vi "DTMF_RealTimeSignalProcessing_Final_COPY.vi"() -> ()   [LabVIEW 2020]
uses:
  <vilib>/Waveform/WDTOps.llb/WDT Index Channel DBL.vi
  <vilib>/Waveform/WDTOps.llb/WDT Get Waveform Subset DBL.vi
  <vilib>/measure/matone.llb/Extract Single Tone Information 1 Chan.vi
  <vilib>/measure/matone.llb/Extract Multiple Tone Information 1 Chan.vi
  <vilib>/measure/NI_MAPro.lvlib
panel:
  out "FFT spectrum - Complete Signal":cluster{"f0":dbl, "df":dbl, "magnitude":dbl[]}(graph)
  in  "Emergency stop":bool
  out "Time Domain Signal - Complete Signal":dbl(graph)
  in  "Bypasing mode - Loop Timer (ms)":u32(knob)=5 scale=0.0..50.0
  out "Case1 - Time Signal":waveform(dbl)(graph)
  out "Case1 - Spectrum":cluster{"f0":dbl, "df":dbl, "magnitude":dbl[]}(graph)
  out "Lower Frequency":T1(array[cluster]) {"detected phase (deg)" format="%_6g"; "detected amplitude" format="%_6p"; "detected frequency" format="%_6f"}
  out "Case1 Subarray Length":dbl
  out "Case1\nTrigger\nStatus":bool
  out "Higher Frequency":T1(array[cluster]) {"detected phase (deg)" format="%_6g"; "detected amplitude" format="%_6p"; "detected frequency" format="%_6f"}
  out "Case0 Subarray Length":dbl
  out "Case0 Start Index":dbl
  out "Time Domain Signal - Detected Button Presses":dbl(graph)
  in  "Scanning mode - Loop Timer (ms)":u32(knob)=5 scale=0.0..50.0
  out "Total Samples(s)":i32
  out "Case1 Start Index":dbl
  out "Case0 - Time Signal":waveform(dbl)(graph)
  out "Case0 - Spectrum":cluster{"f0":dbl, "df":dbl, "magnitude":dbl[]}(graph)
  out "Case0\nTrigger\nStatus":bool
  out "Iteration#":i32
  out "DTMF Number":string
  in  "Select .wav file":path
  # "This program is for the real time processing of the DTMF signals\nPlease adjust the knobs are increasing the scanning speed"
  # "Case - 0 Scanning mode"
  # "Case - 1 Bypassing mode"
  # "Adjust knobs for scanning speed"
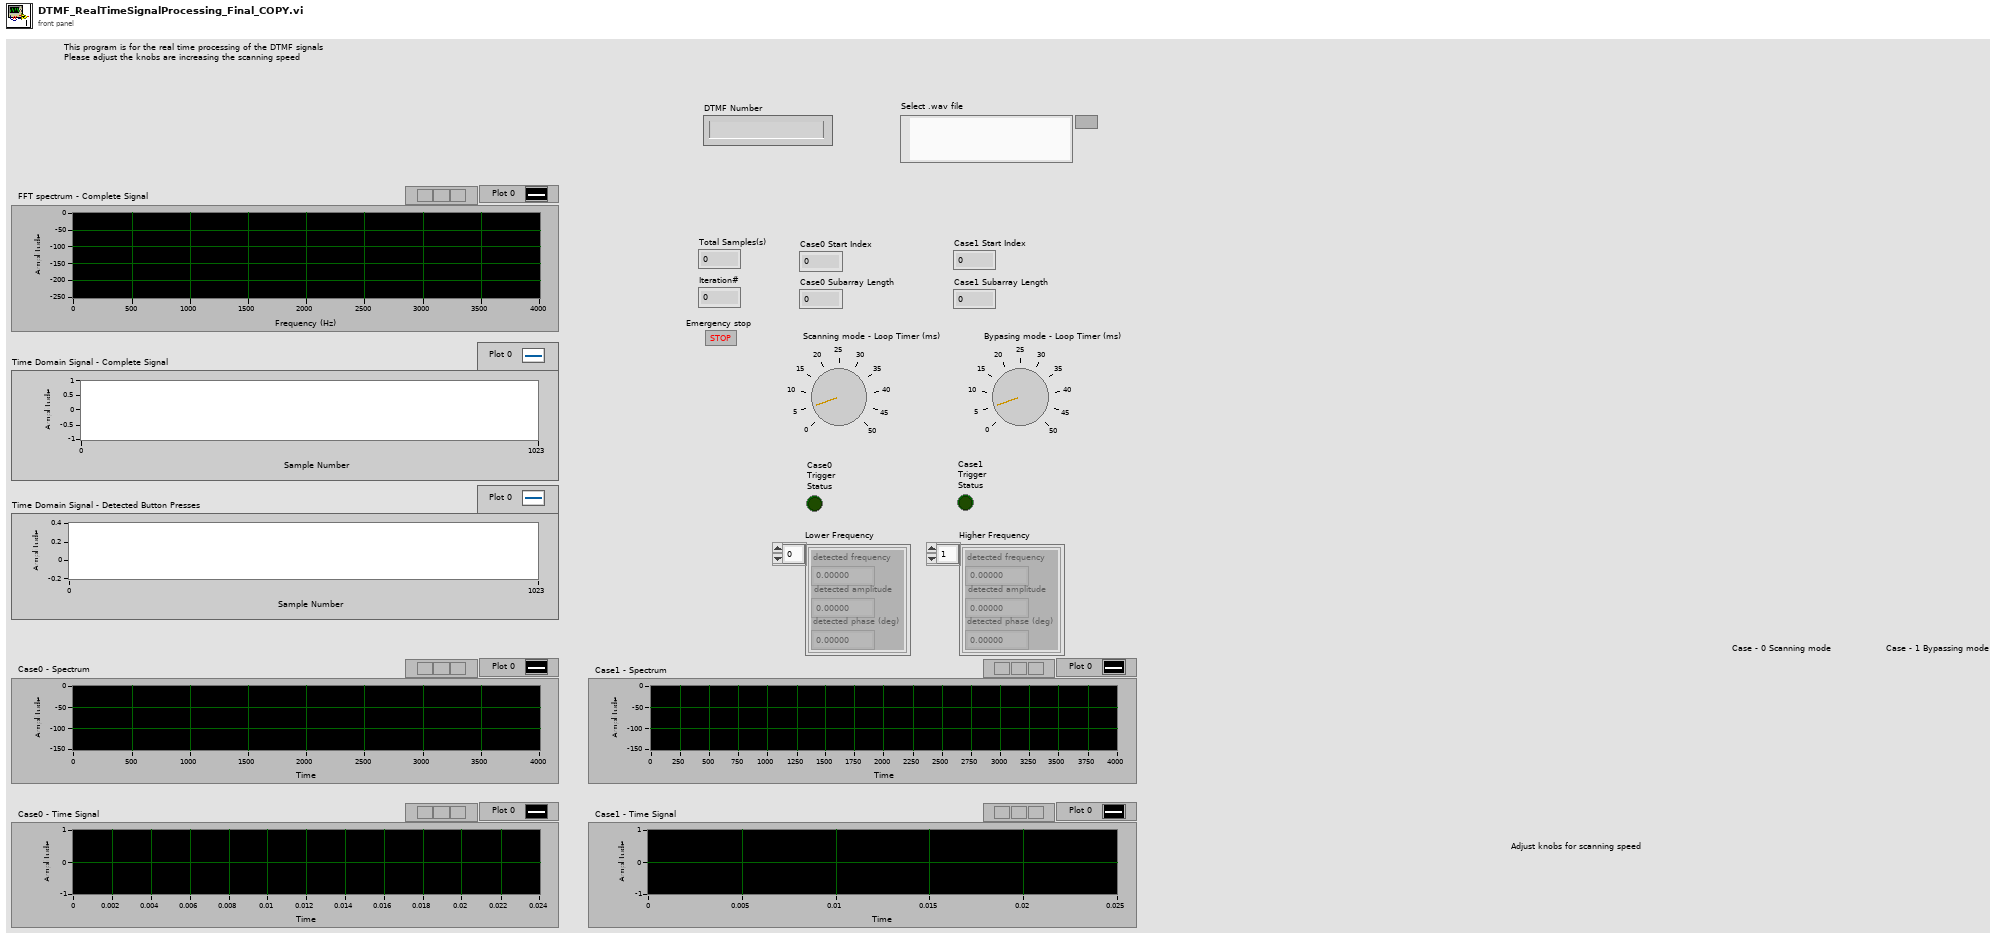
[diagram p1: front panel]
types:
  T1 = cluster{"detected frequency":dbl, "detected amplitude":dbl, "detected phase (deg)":dbl}[]
  T2 = enum32{"none", "input signal", "detected signal", "residual signal"}
  T3 = cluster{"exported time signal":waveform(dbl), "exported spectrum (dB)":cluster{"f0":dbl, "df":dbl, "dB Spectrum (Hann)":dbl[]}}
  T4 = cluster{"f0":dbl, "df":dbl, "dB Spectrum (Hann)":dbl[]}
  T5 = cluster{"detected frequency":dbl, "detected amplitude":dbl, "detected phase (deg)":dbl}
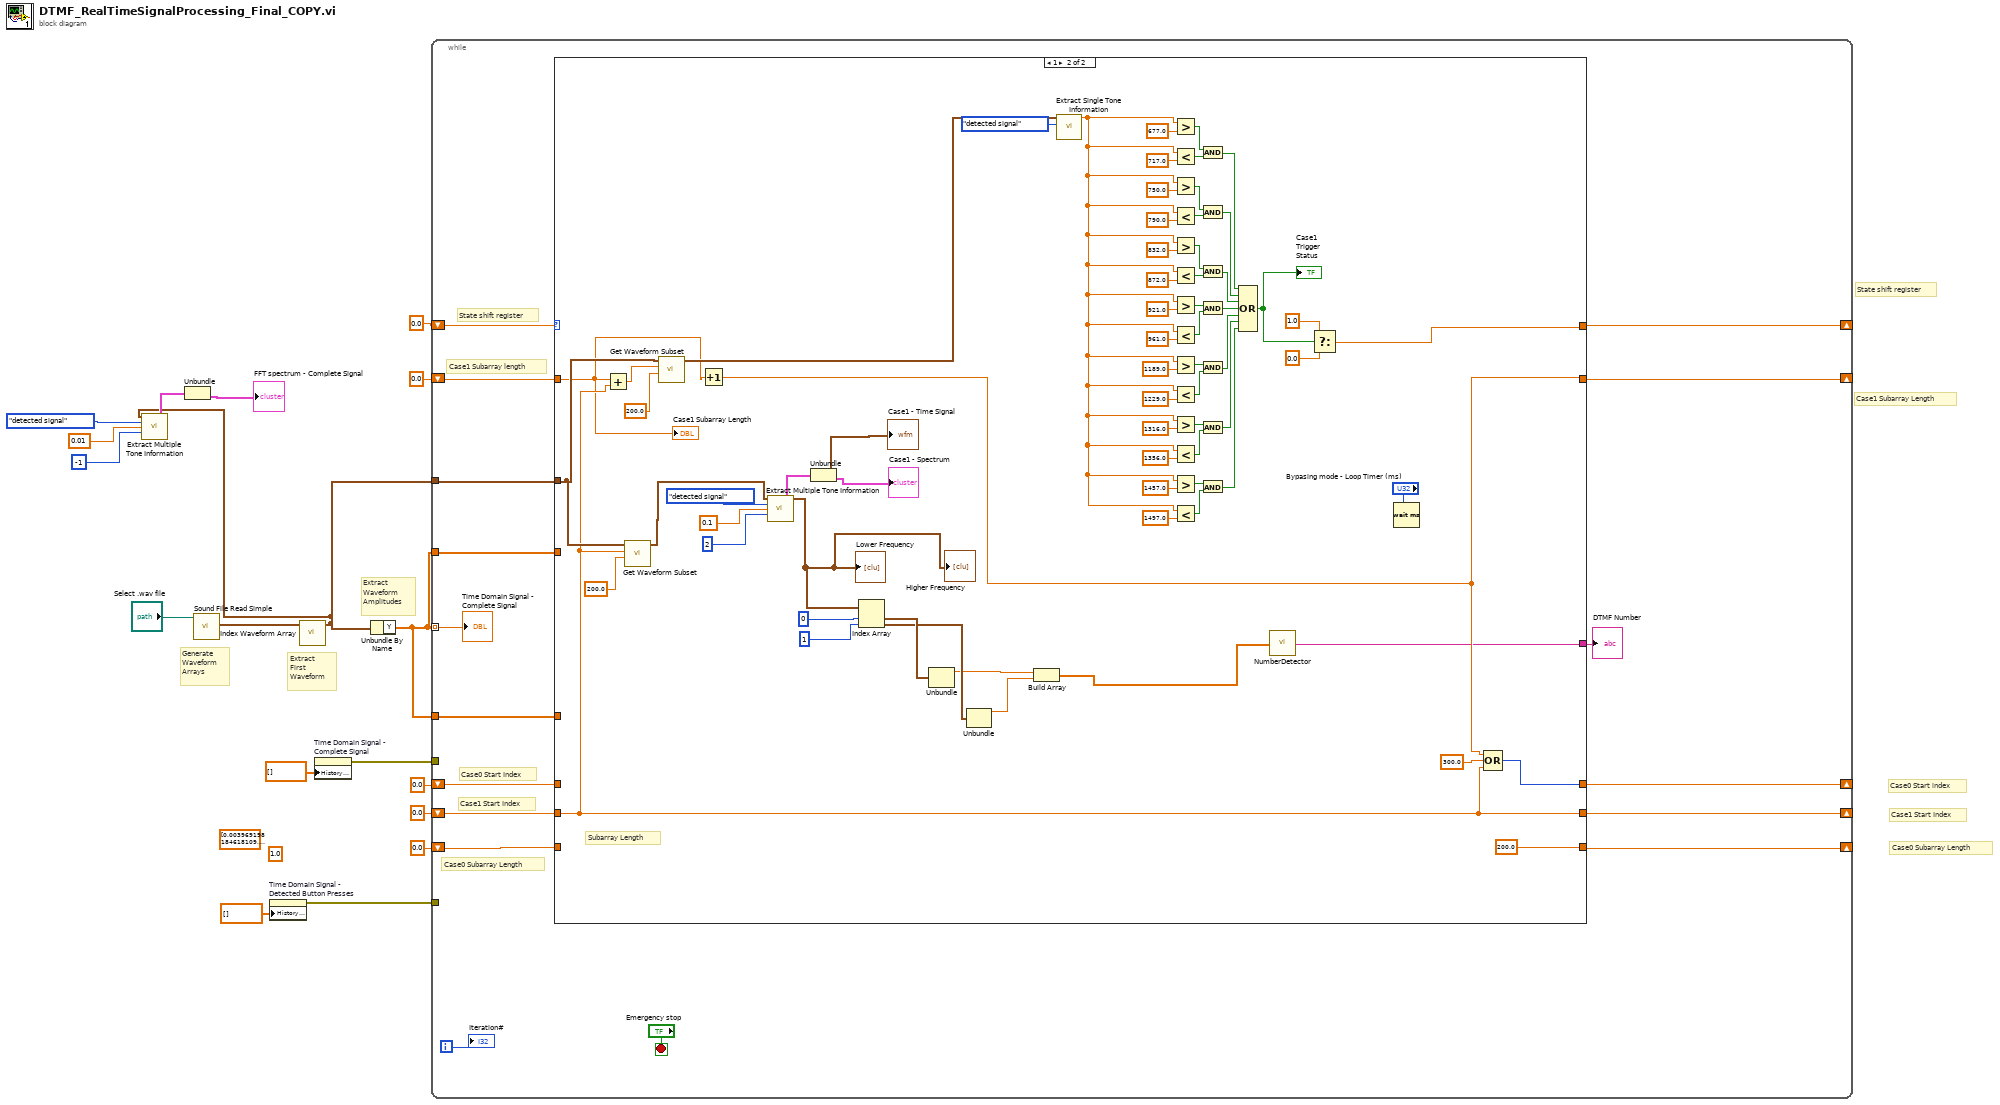
[diagram p0: block diagram]
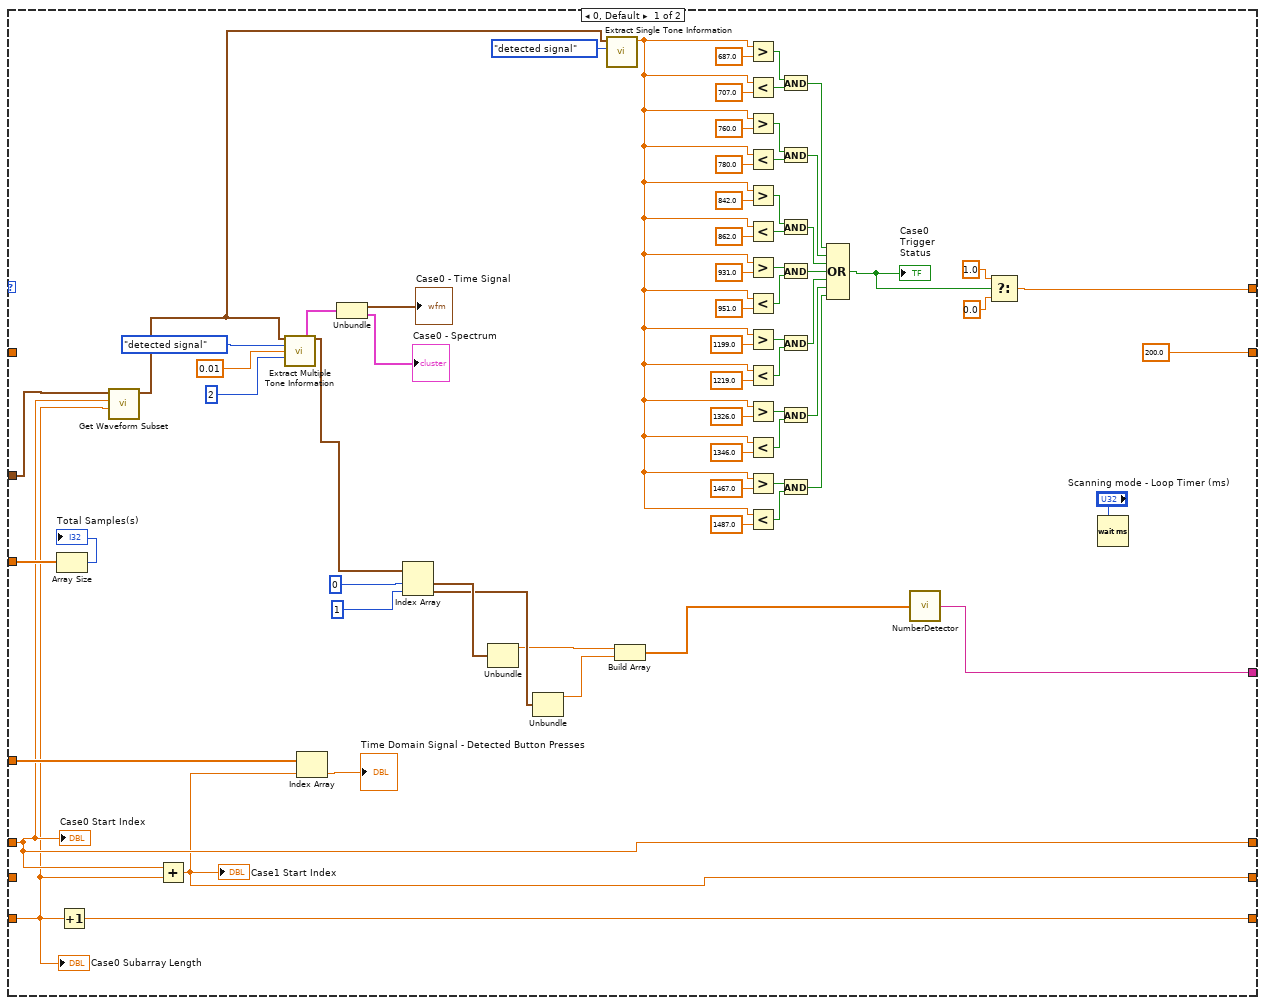
[diagram p2: hidden frame]
diagram:
  (unwired) 1.0 ("X Scale.Offset and Multiplier:Multiplier")
  (unwired) dbl[] [0.003969198184618109, 0.0024133968310094734, 4.40455488561025e-05, 4.448123333843187e-05, 4.502197383414899e-05, 7.105680269600204e-05, 7.300445242572993e-05, 5.6014074009060364e-05, 6.545174464759088e-05, 7.046344706157483e-05, 6.118618513474669e-05, 7.138448410133638e-05, 4.391326300019627e-05, 3.249099587964162e-05, 8.20308269791871e-05, 7.791169449305044e-05, 4.840608842199574e-05, 8.501303350281784e-05, 0.00013087519819616426, 0.0001452090339198192, 0.00015181812473803068, 0.0001410012722641967, 8.606020476188444e-05, 3.4944271796289634e-05, 2.3919549427064746e-05, 2.7074974785822443e-05, 3.9040329870525906e-05, 2.8971216532625324e-05, 5.145508929098338e-05, 5.4916040393555756e-05, 6.0714375869477634e-05, 6.794549159372439e-05, 5.594443118184353e-05, 6.767365554481118e-05, 4.324925112841337e-05, 9.314939094026318e-05, 0.00010865817419412716, 0.00011446621527389493, 0.00014423693570820594, 0.0001460953127618529, 0.00014214107824029505, 0.00011121853908962024, 5.098858703993394e-05, 3.610674914817409e-05, 3.292694288805796e-05, 2.5148267966524824e-05, 6.811399366029676e-05, 7.968819451878582e-05, 7.365538376422848e-05, 7.998768404670619e-05, 9.42775827533405e-05, 0.00010829989168067315, 8.925847194101531e-05, 3.163826956684219e-05, 1.8458412450107225e-05, 2.894333198982863e-05, 5.187008612054176e-05, 5.14781532323922e-05, 4.54032597833059e-05, 4.145585993316444e-05, 4.583967916482741e-05, 5.066810471250756e-05, 5.5432233625921086e-05, 6.672911758409511e-05, 4.842817608719167e-05, 9.415984056234743e-05, 8.647922130734387e-05, 9.110035704959233e-05, 0.00010348109782220863, 0.0001211334395381195, 0.00011335438138589139, 8.957292640500424e-05, 0.0001104703994917259, 9.994009615549219e-05, 9.23972447077788e-05, 6.94264377902343e-05, 5.532891311974586e-05, 4.872993803422138e-05, 4.953239107290117e-05, 5.8018407035194964e-05, 9.127803137437761e-05, 0.00016943044705355632, 0.00015718520615186845, 0.00018757547725267251, 0.00015332349616848623, 0.00014409661719114186, 0.00016884994970799478, 0.00012422099604852496, 0.00011795071019541, 1.9177402465492597e-05, 6.361620869612648e-05, 5.717619361266548e-05, 7.70920783226238e-05, 0.00012079506258917837, 0.0001636691372729251, 0.00019061104114091731, 0.00022286917649631225, 0.00034709098749470497, 0.000360032685246228, 0.00040310830255344335, 0.0003423140334388282, 0.00038592130732406144, 0.00040738913728250906, 0.0003441565749541463, 0.0003547431608808211, 0.00021945600819893356, 0.00018141174759361972, 7.910451295394376e-05, 0.0001009618250945855, 7.564224476842461e-05, 0.00021874642731852035, 0.00042089884070324834, 0.0004974276794532741, 0.000717493571268488, 0.0006640538971434138, 0.000819363042782344, 0.0008628179059320878, 0.0009524353615700349, 0.0010038131175706267, 0.0007750306735778797, 0.0009069872353596249, 0.0006378287012352525, 0.0005052268273016388, 0.0001294351589702371, 0.0003418785794633177, 0.0008011166114727321, 0.001436037121992444, 0.002276865223070367, 0.002838294302796438, 0.0045370419895810424, 0.00517119627638702, 0.007671198160772521, 0.009150440830386323, 0.011951010480551263, 0.015856995547064937, 0.01952446457377027, 0.029294539987389165, 0.04323845260937858, 0.09465296750745547, 0.14238031501891257, 0.1361271615364418, 0.0824222880535919, 0.037831051751406046, 0.02763842751943959, 0.017913478242247174, 0.01541252208037035, 0.010802790803763975, 0.008973050788593716, 0.006992459634290459, 0.0050807219395827795, 0.004289203776573745, 0.0027812463821423527, 0.0022521865775460836, 0.0012532018914398178, 0.0007222655388046516, 0.0002964518148338455, 0.00015320666201682056, 0.00043806273951169203, 0.000610116753015447, 0.0008886387582345324, 0.0007553702875701995, 0.0009547310778193698, 0.0008674793570335321, 0.0009755983823681462, 0.0008576892712847095, 0.0007799959378209144, 0.0007801512734870405, 0.000581046586250408, 0.0005634237737731245, 0.00037688520677899517, 0.00024211017490902682, 0.0001391099453030815, 9.848735854751542e-05, 7.107162676652918e-05, 0.00016711508551520932, 0.0003178050459309747, 0.0003321665039596733, 0.0003795104960579795, 0.00038719817958821735, 0.0004458029666977166, 0.00047209273847857627, 0.0004639332644842537, 0.000374230053293133, 0.0003014849307856567, 0.00038805324915063336, 0.00034296175298586244, 0.0002565923430980299, 0.00011513598924517068, 0.00010110635793627242, 9.833539916328274e-05, 0.00011092000571546677, 3.1468786444658315e-05, 2.981251064249896e-05, 0.00013173595626034308, 0.00019261420108803514, 0.00023462778237111128, 0.0002253613007170444, 0.00030428488403625635, 0.00034329004186024026, 0.0003133470128888824, 0.00030799025993714013, 0.00026215464579647094, 0.0003186586400334151, 0.00026398565762540563, 0.00033603087749758693, 0.00029461864763139, 0.000254077986641385, 0.00015911140496605857, 7.770557625336885e-05, 2.974432618086713e-05, 0.00011377981150248287, 0.000213145695693206, 0.0003064526600948323, 0.0004837274237972076, 0.0005396637322973858, 0.0006925947716733566, 0.0007969827540691752, 0.0008200125546084276, 0.0009512701139103222, 0.0007971080642772455, 0.0009779053881077257, 0.0007630847538956987, 0.0008077386204087759, 0.0006325855977921897, 0.00044724621867851236, 0.0002164414633954468, 0.0002536815307573764, 0.0006745828679373082, 0.0011107383139219503, 0.0021010569801727056, 0.0026761314153702473, 0.003967873360378092, 0.0050526571361386285, 0.006371718019075962, 0.00882813927442431, 0.009986527704078088, 0.014857751109614521, 0.01687450483566293, 0.02567231224777376, 0.03434958759486605, 0.07068516546938654, 0.12777757350430086, 0.14616643757714334, 0.10663103311703657, 0.05072566656583132, 0.030773417512926504, 0.02148894688567684, 0.016084765388888148, 0.013088471009623357, 0.009209951260767383, 0.008171738981921483, 0.005447942659520709, 0.004774384162893179, 0.0031074767882258753, 0.002319109997890845, 0.0015745347052982274, 0.0008087631329511822, 0.0003525168529441314, 9.82115197392905e-05, 0.000462614912594782, 0.0005700575031600617, 0.0009057500776931841, 0.0009096292693389349, 0.0010508880723658581, 0.0010522614128402569, 0.0009171340798170346, 0.0009594764624505156, 0.0007348532732027629, 0.0007778542032069578, 0.0005410947492743702, 0.00043943519657020614, 0.00031540222683018793, 0.00017511136188885546, 0.00011590385711420217, 0.00010979668597776216, 0.00020357428881256388, 0.000265672897960157, 0.00036686053404241906, 0.0003484809996578547, 0.0003737486006566243, 0.0003708252970101547, 0.000368868451048815, 0.00040814518012010953, 0.0003049453829063317, 0.0003114467926072325, 0.00022191281445802102, 0.0001364204323668812, 6.771501770350758e-05, 8.741866570863596e-05, 9.042869464993506e-05, 6.152552274140495e-05, 0.00011468712441402572, 0.0001106935451407812, 0.00012198727743156741, 0.00013390648172357527, 0.00017508755101429613, 0.0002201994740396893, 0.0001545131137876398, 0.0001419668335218303, 0.00013413483662990937, 0.0001650396266657985, 0.00012633705075116206, 0.00013304080030479703, 0.00011280853708597896, 6.20673696017632e-05, 3.993219829715998e-05, 5.236585940469754e-05, 9.163047234890244e-05, 0.00011888175947088787, 0.00014566965377318123, 0.00014562890146144281, 7.730144830645936e-05, 4.167990905243778e-05, 6.210534887433249e-05, 8.517353910534448e-05, 4.308051231562601e-05, 1.70996421311367e-05, 2.7768068171997628e-05, 2.8388298314181795e-05, 8.06011502390716e-05, 0.0001262348668208229, 0.00010873306848589898, 7.097342019992858e-05, 5.52819866314172e-05, 4.847229417194828e-05, 4.946168982124097e-05, 8.704278762220302e-05, 0.00010528365279812353, 9.957941230452963e-05, 8.271448655508176e-05, 4.153907322488169e-05, 1.737059318850597e-05, 4.823848954337302e-05, 6.718034201812235e-05, 7.14955524428289e-05, 7.191780997146302e-05, 7.278623059429391e-05, 4.116697519927217e-05, 2.936605222713053e-05, 7.98040963504798e-05, 9.56032700777792e-05, 0.00013066848763383925, 0.00014568014715674109, 0.00013196371779093321, 7.851223758963966e-05, 1.701291188493292e-05, 6.707967546900085e-05, 5.259791436382229e-05, 5.293609212991933e-05, 6.091667799776681e-05, 5.3706338220212224e-05, 5.437806071779456e-05, 5.591457571628348e-05, 6.0262239528012584e-05, 6.630476522057791e-05, 6.666297508573078e-05, 0.00010545772695758666, 0.00015823985868800169, 0.00013708934824184664, 9.826336319589846e-05, 0.00016890131833910977, 0.00022979410049431937, 0.0002255594896955826, 0.00015716104304215196, 6.852512829012247e-05, 7.77793361984444e-05, 0.00012331085389723518, 0.00011331593631240868, 7.726089563333246e-05, 5.859796408134471e-05, 5.816184572945826e-05, 5.0589317993232264e-05, 3.7680681359289504e-05, 3.156620740206874e-05, 4.070095590154637e-05, 8.723611368613122e-05, 0.00010876778475174031, 0.0001462043241414902, 0.0001680289111337272, 0.00014907642102883812, 0.00013931518123903584, 0.0001328136160759248, 0.00011935816949129191, 6.677036056043265e-05, 1.9279059314653435e-05, 7.346509687274255e-05, 8.423160739861967e-05, 6.397120183258659e-05, 1.6696307102675935e-05, 4.126757544591013e-05, 7.03861994406218e-05, 5.69201164315669e-05, 3.134248388792793e-05, 2.027467715852069e-05, 3.7443511831700714e-05, 5.657627117989812e-05, 6.095917777151183e-05, 8.382612011845038e-05, 9.686492570654583e-05, 8.022879218672187e-05, 6.137763193644651e-05, 7.836551515014601e-05, 9.661681502086106e-05, 0.0001027590771682937, 0.00010072514570094562, 6.46146904032924e-05, 2.191671007220045e-05, 3.789097652818994e-05, 7.512623231232038e-05, 0.00010063869718593082, 9.536401920641791e-05, 7.572683568501372e-05, 6.410952532267226e-05, 6.60566108926513e-05, 6.29298059050159e-05, 6.422272367061009e-05, 7.26850641997581e-05, 7.902279560249476e-05, 0.00010272830355101116, 9.885302499781444e-05, 5.037954593391948e-05, 6.085402608946705e-05, 0.00010576098448856764, 0.00011688134853663606, 9.67727400594962e-05, 9.861144510570926e-05, 9.65238711861668e-05, 6.261642264081396e-05, 2.4793723368062723e-05, 1.0918455156276782e-05, 1.2724147491402633e-05, 2.4716789766694054e-05, 4.222912748631449e-05, 2.840165448980098e-05, 5.936112062045188e-05, 7.511867976478199e-05, 6.001059834158836e-05, 4.645435629141083e-05, 2.162004076828713e-05, 2.9715175207040688e-05, 7.262979131781553e-05, 8.543030542784143e-05, 7.118350267507755e-05, 2.6726415063257925e-05, 5.328211101427645e-05, 8.42980020178332e-05, 8.368163728544642e-05, 6.70840811591894e-05, 4.362379784220743e-05, 3.8217199156709946e-05, 4.348764864132397e-05, 4.626162258513739e-05, 4.804100758189643e-05, 4.054110044048473e-05, 3.0440476828512828e-05, 2.3351897841079655e-05, 2.6648475959068e-05, 6.009892038118268e-05, 7.827462275710724e-05, 7.347510305028777e-05, 5.285307869094695e-05, 2.7031310629625442e-05, 2.8911334736324906e-05, 4.654419937728862e-05, 4.8250486403781965e-05, 4.252536896292137e-05, 4.748350574663552e-05, 4.592224491202041e-05, 3.890711092981841e-05, 4.280602312040083e-05, 6.262684324694968e-05, 8.046840211509612e-05, 8.489377488692691e-05, 6.279209656072767e-05, 3.764639496486363e-05, 4.087789563316127e-05, 2.8082890960629245e-05, 1.6754922224207566e-05, 4.526250839066248e-05, 8.450110696062193e-05, 9.081864879792681e-05, 6.787045825835487e-05, 7.774044800297394e-05, 8.077195160744638e-05, 5.027853710722988e-05, 5.96694032622772e-05, 5.9437514694410105e-05, 5.3000470297082725e-05, 8.125342524469679e-05, 0.00012339642499246574, 0.00013593362881769158, 0.00011087373454206096, 8.060879872117106e-05, 5.85241194035258e-05, 7.59668392251561e-05, 0.00011742367041904182, 0.0001377418152846472, 0.00012676189080436346, 0.00010424746164400893, 9.729601045909138e-05, 0.00010866127245498176, 0.00011253103848342785, 9.194104187393223e-05, 5.308479077347102e-05, 1.8055844865154087e-05, 3.4161791333147285e-05, 4.2783773770306305e-05, 2.7366315328394843e-05, 6.452997976515523e-05, 0.0001149276328202564, 0.00011154519381355821, 6.372246781003783e-05, 4.1173326027605135e-05, 4.185376526941851e-05, 5.752028468544232e-05, 6.056816822111249e-05, 4.35446181035797e-05, 4.2562476912272006e-05, 4.4734983617018357e-05, 6.568776700146115e-05, 7.753085203140569e-05, 7.871192839326796e-05, 8.352341948471912e-05, 7.569279155459991e-05, 5.282238618556747e-05, 3.873488585625387e-05, 2.8279967730156163e-05, 1.6773797926476347e-05, 3.308435346184758e-05, 5.4276495663436795e-05, 5.237207141049904e-05, 2.959862669854432e-05, 9.49736427069395e-06, 3.184825077826278e-05, 5.851923576567817e-05, 5.158366481291845e-05, 1.0867552082891716e-05, 5.0054347618526174e-05, 7.287770396468634e-05, 5.099999849221781e-05, 3.772712357308911e-05, 7.742865900523118e-05, 8.636623987488972e-05, 6.4155884384612e-05, 3.710827391146563e-05, 1.4483083410430621e-05, 3.725649875385264e-05, 6.59301501990798e-05, 8.597385459661695e-05, 8.427297533381409e-05, 5.977088288028281e-05, 4.3588253002989764e-05, 4.6802369929505624e-05, 4.908365645617985e-05, 2.8010016888260092e-05, 6.739535192131295e-05, 0.00010535096441503566, 7.226167652604903e-05, 1.0914342316929139e-05, 1.561905649780243e-05, 3.94988401696506e-05, 5.534971744840786e-05, 3.266276410670713e-05, 1.7057400754071163e-05, 2.7433992223310198e-05, 2.185645540292438e-05, 9.349338804130616e-06, 8.421346482703344e-06, 2.7191957447498916e-05, 4.912790477642461e-05, 4.871300335954871e-05, 4.028747084245908e-05, 3.535606989710528e-05, 3.7883075665190865e-05, 5.393480656789241e-05, 7.15153090096189e-05, 7.30892239420983e-05, 5.682372696702926e-05, 3.290744934159215e-05, 1.8005886041082607e-05, 2.372446175328017e-05, 2.8191377878069782e-05, 4.456772911427592e-05, 4.102159118051863e-05, 3.648915200659934e-05, 5.646758660091236e-05, 8.333853260554697e-05, 8.356478462646534e-05, 4.644812281479802e-05, 4.0057994885683845e-05, 7.14895307344592e-05, 7.520110640679237e-05, 6.846198774484605e-05, 5.26567242329375e-05, 1.3086292620349404e-05, 3.180240816395685e-05, 5.595735536504747e-05, 5.210585628750412e-05, 4.9432249260157664e-05, 9.994356815597617e-05, 0.00012424619453367544, 0.00010303690217528854, 7.253534191794038e-05, 5.736591360840302e-05, 3.5929854871557584e-05, 1.6939941268118602e-05, 6.405206090923974e-05, 8.470717979899605e-05, 6.64826737938609e-05, 5.752573027042049e-05, 6.810688536894389e-05, 7.27856018098631e-05, 5.7348753968740794e-05, 4.842226074777694e-05, 9.154993558243549e-05, 0.00010653373402428958, 8.897524372418692e-05, 6.948519654460094e-05, 7.061972495983032e-05, 8.29416429378298e-05, 9.031751097491205e-05, 8.119524409072753e-05, 5.164766392825825e-05, 5.840693659810795e-05, 6.946776572105235e-05, 7.699580218257649e-05, 8.558459469263746e-05, 5.667639185622447e-05, 3.058033081101322e-05, 3.485558396072937e-05, 1.0930226612758517e-05, 3.483855057192427e-05, 5.324897501979144e-05, 3.902554354624459e-05, 3.224124680965142e-05, 5.3171097079913366e-05, 6.03678257386858e-05, 5.923285876803141e-05, 7.03857261575969e-05, 8.848646029002045e-05, 7.918293611269923e-05, 2.2148667313176568e-05, 4.926292208454908e-05, 7.186605625069713e-05, 4.648387467613763e-05, 3.8902540687510085e-05, 1.7999540189644502e-05, 2.6564474398104183e-05, 5.038313442628017e-05, 5.8737751462507106e-05, 8.648232179694932e-05, 0.00010873630844857533, 9.563181288365165e-05, 6.44238212944706e-05, 6.379854992321045e-05, 6.17084064098262e-05, 5.215235243182937e-05, 5.375314156446913e-05, 4.343136463676183e-05, 3.247153710290878e-05, 2.2521970794115682e-05, 1.9044652950477272e-05, 4.2856288951552394e-05, 8.392096968973451e-05, 9.576377922032171e-05, 7.289683842092148e-05, 7.426800958555215e-05, 5.641019833563324e-05, 3.5650845974023675e-05, 6.606776089388405e-05, 6.849820166371782e-05, 4.503828232132285e-05, 7.029659011502802e-05, 8.469533980502242e-05, 4.561113746997961e-05, 6.93237025682427e-05, 6.911410313253096e-05, 2.8242510927376296e-05, 3.6818404316679e-05, 5.031021397706077e-05, 4.629192789877277e-05, 1.263909213226551e-05, 3.742124797535805e-05, 7.954025154695315e-05, 8.738096055071372e-05, 7.952224633678165e-05, 7.475725641429231e-05, 3.5137130028020475e-05, 7.081718794851545e-06, 2.4845474136509524e-05, 7.216673965156714e-05, 8.484377272538738e-05, 5.229616632754635e-05, 2.0385436033542022e-05, 5.472640904063822e-06, 1.164426233182113e-05, 2.2827404524546056e-05, 6.537405827079216e-05, 8.9958938183218e-05, 8.62942169750996e-05, 4.353239189753934e-05, 1.538486494552081e-05, 4.951743751279212e-05, 5.360952721819399e-05, 3.942455810687565e-05, 3.31194578301596e-05, 3.093204554623581e-05, 3.656652912003321e-05, 4.1977083819938405e-05, 2.4730117084454208e-05, 8.261120120505278e-06, 1.685053128476759e-05, 2.9049097434372693e-05, 1.692075484575048e-05, 4.165821351617546e-06, 4.158266677454387e-05, 0.00010373023171590118, 0.00012426723364965521, 9.804294767965362e-05, 9.102398675908579e-05, 9.920772711437317e-05, 8.567933089088223e-05, 6.524810336300054e-05, 6.0395599228716574e-05, 7.344747583576106e-05, 8.856838930786096e-05, 9.485170689979115e-05, 9.412507844453843e-05, 7.71087329025092e-05, 3.651596209937633e-05, 3.394414579574172e-05, 6.0539667091931e-05, 6.162473851427232e-05, 4.7250154592393205e-05, 5.262447485581156e-05, 5.6852103368508344e-05, 5.1277471664516685e-05, 6.278104659585434e-05, 8.59006723247007e-05, 0.00010161313996869728, 0.00010199292107761546, 0.0001084431069429474, 9.448465210481588e-05, 5.153196143447218e-05, 2.5517018468356046e-05, 4.992635630791478e-05, 6.952199912881514e-05, 5.869047181336314e-05, 3.0975980392916624e-05, 1.665115009658699e-05, 2.999561394080758e-05, 6.538492531160737e-05, 8.531609215836886e-05, 7.065349266065556e-05, 5.527978841831917e-05, 3.281423588334988e-05, 3.399738101841561e-05, 7.419779433165999e-05, 7.092466954814642e-05, 6.821962695287773e-05, 0.00011826132145292387, 0.00011356770165259288, 8.748292122287419e-05, 8.211124481887207e-05, 4.950537826506543e-05, 1.9892712019559078e-05, 4.775630620546596e-05, 5.1927451970792084e-05, 7.040024695823356e-05, 0.00012191886368228995, 0.000131057739648167, 0.00010295386071494058, 6.256159179971039e-05, 3.536348557499907e-05, 1.636231514078733e-05, 2.01545329894574e-05, 4.630496381523116e-05, 4.615298716116953e-05, 2.3989655431292977e-05, 1.7817879564334736e-05, 3.925426696654823e-05, 5.317698069858208e-05, 6.115679218266108e-05, 3.882301545855975e-05, 2.767247586463203e-05, 7.6807873156604e-05, 9.190368299501447e-05, 8.949854235652135e-05, 9.283280254061955e-05, 8.971537645524053e-05, 6.52931675847153e-05, 4.0362876037288505e-05, 3.668906062515573e-05, 3.188444053977858e-05, 7.090527826553477e-05, 7.89789778581111e-05, 0.00010895948832953836, 0.00010863237192899123, 7.047714301162298e-05, 8.197169901706302e-05] ("FFT Spectrum")
  # "Case1 Subarray Length"
  # "Case0 Subarray Length"
  # "Case1 Start Index"
  # "Case0 Start index"
  # "State shift register"
  # "Extract\nWaveform\nAmplitudes"
  # "Extract\nFirst\nWaveform"
  # "Generate\nWaveform\nArrays"
  n1 = call <vilib>:"Sound File Read Simple.vi"("path"="Select .wav file") -> ("data"=w17:waveform(dbl)[])  [unwired: 7 in, 3 out]
  n2 = property on="Time Domain Signal - Detected Button Presses" class="WFChart (strict)"("History Data"=dbl[] []) -> (error out=w11:errorcluster)  [unwired: 2 in, 1 out]
  n3 = call-poly <vilib>:"Index Waveform Array.vi"("waveform array"=w17) -> ("waveform"=w1:waveform(dbl))  [unwired: 9 in, 1 out]
  n4 = call-poly <vilib>:"Extract Multiple Tone Information.vi"("time signal in"=w1, "export mode"=T2."detected signal", "threshold"=0.01, "max num tones"=-1) -> ("exported signals"=w3:T3)  [unwired: 9 in, 2 out]
  n5 = Unbundle(w3) -> ("exported spectrum (dB)"=→"FFT spectrum - Complete Signal":T4)  [unwired: 1 out]
  n6 = property on="Time Domain Signal - Complete Signal" class="WFChart (strict)"("History Data"=dbl[] []) -> (error out=w16:errorcluster)  [unwired: 2 in, 1 out]
  n7 = Unbundle By Name(w1) -> ("Y"=w9:dbl[])
  n8 = while {
    tunnel: w9 -> [w34] mode=indexing
    tunnel: w16 -> [_]
    shift-right: [w33] -> _
    shift-left: 0.0 -> [w32]
    shift-right: [w30] -> _
    shift-left: 0.0 ("f") -> [w29]
    shift-right: [w28] -> _
    shift-left: 0.0 -> [w21]
    tunnel: w9 -> [w27]
    tunnel: w11 -> [_]
    tunnel: w9 -> [w26]
    tunnel: w1 -> [w25]
    shift-right: [w24] -> _
    shift-left: 0.0 -> [w20]
    shift-right: [w22] -> _
    shift-left: 0.0 -> [w23]
    i -> [w31]
    stop <- "Emergency stop" stop-if-true
    # "State shift register"
    # "Case1 Start Index"
    # "Case1 Subarray length"
    # "Case0 Start Index"
    # "Case0 Subarray Length"
    n9 = case shown="1" w29 {
      tunnel: [w101 200.0] -> w33
      tunnel: w32 -> [w45 _]
      tunnel: [w95 w170] -> w30
      tunnel: w21 -> [w48 _]
      tunnel: [w48 w115] -> w28
      tunnel: w27 -> [w100 _]
      tunnel: w26 -> [w96 _]
      tunnel: w25 -> [w88 w159]
      tunnel: [w47 w116] -> w24
      tunnel: w23 -> [_ w113]
      tunnel: [200.0 w117] -> w22
      tunnel: w20 -> [_ w116]
      tunnel: [w36 w105] -> w19
      frame 0, Default {
        n10 = Array Size(array=w96) -> (size(s)=→"Total Samples(s)":i32)
        n11 = Increment(x=w45) -> (x+1=w101:dbl)
        n12 = call-poly <vilib>:"Get Waveform Subset.vi"("duration"=w45, "start samples/time"=w48, "waveform in"=w88) -> ("waveform out"=w87:waveform(dbl))  [unwired: 3 in, 3 out]
        n13 = Add(x=w48, y=w45) -> (x+y=w47:dbl)
        "Case1 Start Index" <- w47
        n14 = call-poly <vilib>:"Extract Multiple Tone Information.vi"("time signal in"=w87, "export mode"=T2."detected signal", "threshold"=0.01, "max num tones"=2) -> ("exported signals"=w91:T3, "multiple tone information"=w38:T1)  [unwired: 9 in, 1 out]
        n15 = Index Array(array=w100, index=w47) -> (element=→"Time Domain Signal - Detected Button Presses":dbl)
        n16 = Unbundle(w91) -> ("exported time signal"=→"Case0 - Time Signal":waveform(dbl), "exported spectrum (dB)"=→"Case0 - Spectrum":T4)
        n17 = Index Array(array=w38, index #1=0 ("index"), index #2=1 ("index")) -> (element #1=w43:T5, element #2=w41:T5)
        n18 = Unbundle(w43) -> ("detected frequency"=w40:dbl)  [unwired: 2 out]
        n19 = Unbundle(w41) -> ("detected frequency"=w39:dbl)  [unwired: 2 out]
        n20 = call-poly <vilib>:"Extract Single Tone Information.vi"("export mode"=T2."detected signal", "time signal in"=w87) -> ("detected frequency"=w50:dbl)  [unwired: 4 in, 5 out]
        n21 = Build Array(w40, w39) -> (w37:dbl[])
        n22 = Greater?(x=w50, y=687.0) -> (0:w83:bool)
        n23 = Less?(x=w50, y=707.0) -> (x < y?=w82:bool)
        n24 = Greater?(x=w50, y=760.0) -> (0:w79:bool)
        n25 = Less?(x=w50, y=780.0) -> (x < y?=w78:bool)
        n26 = Greater?(x=w50, y=842.0) -> (0:w75:bool)
        n27 = Less?(x=w50, y=862.0) -> (x < y?=w74:bool)
        n28 = Greater?(x=w50, y=931.0) -> (0:w71:bool)
        n29 = Less?(x=w50, y=951.0) -> (x < y?=w70:bool)
        n30 = Greater?(x=w50, y=1199.0) -> (0:w67:bool)
        n31 = Less?(x=w50, y=1219.0) -> (x < y?=w66:bool)
        n32 = Greater?(x=w50, y=1326.0) -> (0:w63:bool)
        n33 = Less?(x=w50, y=1346.0) -> (x < y?=w62:bool)
        n34 = Greater?(x=w50, y=1467.0) -> (0:w60:bool)
        n35 = Less?(x=w50, y=1487.0) -> (x < y?=w61:bool)
        n36 = And(x=w83, y=w82) -> (x .and. y?=w57:bool)
        n37 = And(x=w79, y=w78) -> (x .and. y?=w56:bool)
        n38 = And(x=w75, y=w74) -> (x .and. y?=w55:bool)
        n39 = And(x=w71, y=w70) -> (x .and. y?=w54:bool)
        n40 = And(x=w67, y=w66) -> (x .and. y?=w53:bool)
        n41 = And(x=w63, y=w62) -> (x .and. y?=w52:bool)
        n42 = And(x=w60, y=w61) -> (x .and. y?=w51:bool)
        n43 = Compound Arithmetic op=OR(w57, w56, w55, w54, w53, w52, w51) -> (w49:bool)
        "Case0\nTrigger\nStatus" <- w49
        n44 = call "NumberDetector.vi"("Array"=w37) -> ("f"=w36:string)
        n45 = Select(t=1.0, s=w49, f=0.0) -> (s? t:f=w95:dbl)
        n46 = Wait (ms)(milliseconds to wait="Scanning mode - Loop Timer (ms)") -> ()  [unwired: 1 out]
        "Case0 Subarray Length" <- w45
        "Case0 Start Index" <- w48
      }
      frame 1 {
        # "Subarray Length"
        n47 = Add(x=w113, y=w116) -> (x+y=w119:dbl)
        n48 = call-poly <vilib>:"Get Waveform Subset.vi"("duration"=200.0, "start samples/time"=w116, "waveform in"=w159) -> ("waveform out"=w161:waveform(dbl))  [unwired: 3 in, 3 out]
        n49 = call-poly <vilib>:"Get Waveform Subset.vi"("duration"=200.0, "start samples/time"=w119, "waveform in"=w159) -> ("waveform out"=w121:waveform(dbl))  [unwired: 3 in, 3 out]
        n50 = Increment(x=w113) -> (x+1=w117:dbl)
        n51 = call-poly <vilib>:"Extract Multiple Tone Information.vi"("time signal in"=w161, "export mode"=T2."detected signal", "threshold"=0.1, "max num tones"=2) -> ("exported signals"=w164:T3, "multiple tone information"=w104:T1)  [unwired: 9 in, 1 out]
        "Lower Frequency" <- w104
        "Higher Frequency" <- w104
        n52 = Unbundle(w164) -> ("exported time signal"=→"Case1 - Time Signal":waveform(dbl), "exported spectrum (dB)"=→"Case1 - Spectrum":T4)
        n53 = Index Array(array=w104, index #1=0 ("index"), index #2=1 ("index")) -> (element #1=w111:T5, element #2=w109:T5)
        n54 = Unbundle(w111) -> ("detected frequency"=w108:dbl)  [unwired: 2 out]
        n55 = Unbundle(w109) -> ("detected frequency"=w107:dbl)  [unwired: 2 out]
        n56 = Build Array(w108, w107) -> (w106:dbl[])
        n57 = call-poly <vilib>:"Extract Single Tone Information.vi"("export mode"=T2."detected signal", "time signal in"=w121) -> ("detected frequency"=w122:dbl)  [unwired: 4 in, 5 out]
        n58 = Greater?(x=w122, y=677.0) -> (0:w155:bool)
        n59 = Less?(x=w122, y=717.0) -> (x < y?=w154:bool)
        n60 = Greater?(x=w122, y=750.0) -> (0:w151:bool)
        n61 = Less?(x=w122, y=790.0) -> (x < y?=w150:bool)
        n62 = Greater?(x=w122, y=832.0) -> (0:w147:bool)
        n63 = Less?(x=w122, y=872.0) -> (x < y?=w146:bool)
        n64 = Greater?(x=w122, y=921.0) -> (0:w143:bool)
        n65 = Less?(x=w122, y=961.0) -> (x < y?=w142:bool)
        n66 = Greater?(x=w122, y=1189.0) -> (0:w139:bool)
        n67 = Less?(x=w122, y=1229.0) -> (x < y?=w138:bool)
        n68 = Greater?(x=w122, y=1316.0) -> (0:w135:bool)
        n69 = Less?(x=w122, y=1356.0) -> (x < y?=w134:bool)
        n70 = Greater?(x=w122, y=1457.0) -> (0:w132:bool)
        n71 = Less?(x=w122, y=1497.0) -> (x < y?=w133:bool)
        n72 = And(x=w155, y=w154) -> (x .and. y?=w129:bool)
        n73 = And(x=w151, y=w150) -> (x .and. y?=w128:bool)
        n74 = And(x=w147, y=w146) -> (x .and. y?=w127:bool)
        n75 = And(x=w143, y=w142) -> (x .and. y?=w126:bool)
        n76 = And(x=w139, y=w138) -> (x .and. y?=w125:bool)
        n77 = And(x=w135, y=w134) -> (x .and. y?=w124:bool)
        n78 = And(x=w132, y=w133) -> (x .and. y?=w123:bool)
        n79 = Compound Arithmetic op=OR(w129, w128, w127, w126, w125, w124, w123) -> (w120:bool)
        "Case1\nTrigger\nStatus" <- w120
        n80 = call "NumberDetector.vi"("Array"=w106) -> ("f"=w105:string)
        n81 = Select(t=1.0, s=w120, f=0.0) -> (s? t:f=w170:dbl)
        n82 = Wait (ms)(milliseconds to wait="Bypasing mode - Loop Timer (ms)") -> ()  [unwired: 1 out]
        n83 = Compound Arithmetic op=OR(w117, 300.0 ("value"), w116) -> (w115:i32)
        "Case1 Subarray Length" <- w113
      }
    }
    "DTMF Number" <- w19
    "Time Domain Signal - Complete Signal" <- w34
    "Iteration#" <- w31
  }
